vi "ztrmv - Triangle Matrix-Vector Product (CDB).vi"(4 "diagonal":T2 items=["Non-unit", "Unit"], 7 "operation A":T3 items=["Direct", "Conjugated & Transposed", "Transposed"], 8 "matrix A type":T1=3 items=["Lower Triangular"=2, "Upper Triangular"=3], 10 "x":cdb[](array[numeric]), 11 "A":T4) -> (0 "error":i32, 3 "ztrmv":cdb[](array[numeric]))   [LabVIEW 2018, in "NI_AALBLAS.lvlib"]
doc: "Calculates the product of a triangular matrix and a vector."
uses:
  NI_AALBLAS.lvlib
  ComplexMatrix.ctl
  LV_Transpose.ctl
  LV_Diag.ctl
  LV_UpLo.ctl
  Order.ctl
  Fucntion.ctl
  BLAS2 Utility(CDB).vi
  NI_Matrix.lvlib
panel:
  # "ztrmv=op(A)*x"
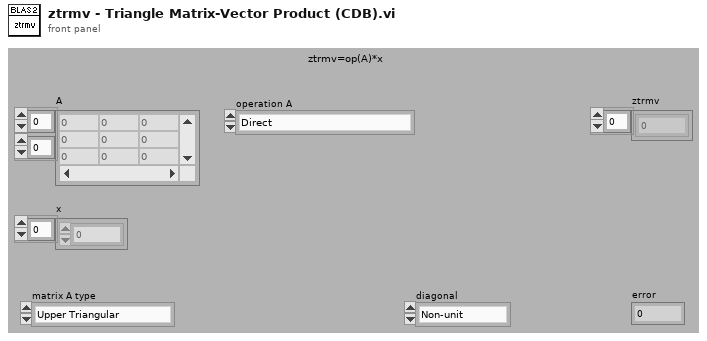
[diagram p1: front panel]
types:
  T1 = typedef "NI_AALBLAS.lvlib/LV_UpLo.ctl" = i32
  T2 = typedef "NI_AALBLAS.lvlib/LV_Diag.ctl" = i32
  T3 = typedef "NI_AALBLAS.lvlib/LV_Transpose.ctl" = i32
  T4 = typedef "NI_Matrix.lvlib/ComplexMatrix.ctl" = cdb[][]
  T5 = typedef "NI_AALBLAS.lvlib/Fucntion.ctl" = u16
  T6 = typedef "NI_AALBLAS.lvlib/Order.ctl" = i32
  T7 = typedef "NI_AALBLAS.lvlib/Diag.ctl" = i32
  T8 = typedef "NI_AALBLAS.lvlib/Operation_Transpose.ctl" = i32
  T9 = typedef "NI_AALBLAS.lvlib/UpLo.ctl" = i32
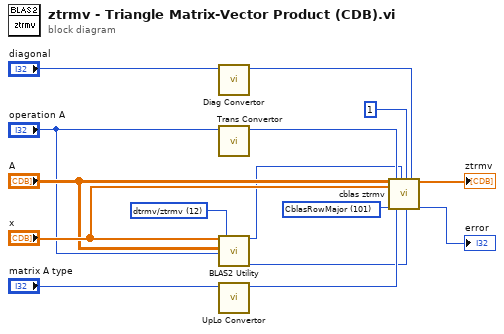
[diagram p0: block diagram]
diagram:
  w1 = T5 12 items=["ddot/zdotu/zdotc", "daxpy/zaxpy", "dnrm2/dznrm2", "dasum/dzasum", "dcopy/zcopy", "dswap/zswap", "drotm", "drot/zdrot", "idamax/izamax", "idamin/izamin", "dgemv/zgemv", "dsymv/zhemv", "dtrmv/ztrmv", "dsyr/zher", "dsyr2/zher2", "dger/zgeru/zgerc", "dtrsv/ztrsv", "dgemm/zgemm", "dsymm/zsymm/zhemm", "dtrmm/ztrmm", "dsyrk/zsyrk/zherk", "dsyr2k/zsyr2k/zher2k", "dtrsm/ztrsm"] ("function")
  w8 = T6 101 items=["CblasRowMajor"=101, "CblasColMajor"=102] ("order")
  n1 = call "Diag Convertor.vi"("diagonal"="diagonal") -> ("diag"=w12:T7)  [unwired: 10 out]
  n2 = call "Trans Convertor.vi"("operation"="operation A") -> ("trans"=w11:T8)  [unwired: 10 out]
  n3 = call-poly "BLAS2 Utility.vi"("x"="x", "A"="A", "operation A"="operation A", "function"=w1) -> ("lda"=w3:i32, "n"=w2:i32)  [unwired: 1 in, 13 out]
  n4 = call "UpLo Convertor.vi"("triangle matrix type"="matrix A type") -> ("uplo"=w14:T9)  [unwired: 10 out]
  n5 = call "cblas ztrmv.vi"("A"="A", "x"="x", "order"=w8, "transA"=w11, "uplo"=w14, "lda"=w3, "incx"=1 ("incX"), "n"=w2, "diag"=w12) -> ("ztrmv"=→"ztrmv":cdb[], "error"=→"error":i32)  [unwired: 9 out]
